vi "Pulse_Period_Measurement.vi"() -> ()   [LabVIEW 2019]
uses:
  <vilib>/Platform/TimedLoop/XDataNode/timing_clust.ctl
  <vilib>/Platform/TimedLoop/XDataNode/nitl_modes.ctl
  <vilib>/Platform/TimedLoop/XDataNode/wakeup.ctl
  <vilib>/rvi/Emulation/niFpgaSctlEmulationGetInTimedLoop.vi
  <vilib>/rvi/Emulation/niFpgaEmulationReportErrorSimple.vi
  <vilib>/rvi/Emulation/niFpgaGetClockAttributes.vi
  <vilib>/rvi/Emulation/niFpgaCriticalErrorInLSC.vi
  <vilib>/rvi/eio/common/nirviEmuTemplateMethod_errors.vi
  <vilib>/platform/TimedLoop/XDataNode/XDataNode.xnode
  <vilib>/eio/EIONode/EIONode.xnode
  <vilib>/Platform/TimedLoop/XDataNode/XDNodeRunTimeDep.lvlib
panel:
  out "DIO3_MODE_SWITCH":u32
  out "DIO2_ON_OFF_SWITCH":u32
  out "DIO1_R_THROTTLE":u32
  out "DIO0_L_THROTTLE":u32
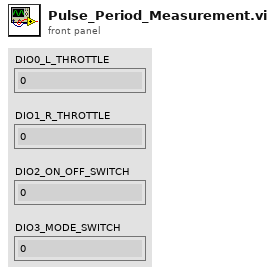
[diagram p1: front panel]
types:
  T1 = typedef "XDNodeRunTimeDep.lvlib/timing_clust.ctl" = cluster{"Expected End [f-1]":u64, "Actual End [f-1]":u64, "Finished Late? [f-1]":bool, "Expected End [i-1]":u64, "Actual End [i-1]":u64, "Finished Late? [i-1]":bool, "Expected Start [i]":u64, "Actual Start [i]":u64, "Expected Start [f]":u64, "Actual Start [f]":u64, "Source Name":string, "Structure Name":string, "Period":i64, "Deadline":i64, "Offset":i64, "Start":i64, "Priority":i32, "Timeout":i32, "Mode":T2, "Wakeup Reason":T3, "Error":errorcluster, "Source Type":string, "Secondary Source Type":string, "Global End Time":u64, "Global Start Time":u64, "Frame Duration":u64, "Iteration Duration":u64, "Assigned CPU":i32, "I/O Scan Engine Mode":u32}
  T2 = typedef "XDNodeRunTimeDep.lvlib/nitl_modes.ctl" = enum32{"No Change", "Process missed periods, maintain original phase", "Discard missed periods, maintain original phase", "Process missed periods, ignore original phase", "Discard missed periods, ignore original phase"}
  T3 = typedef "XDNodeRunTimeDep.lvlib/wakeup.ctl" = enum32{"Normal", "Aborted", "Asynchronous wakeup", "Timing source error", "Timed loop error", "Timeout"}
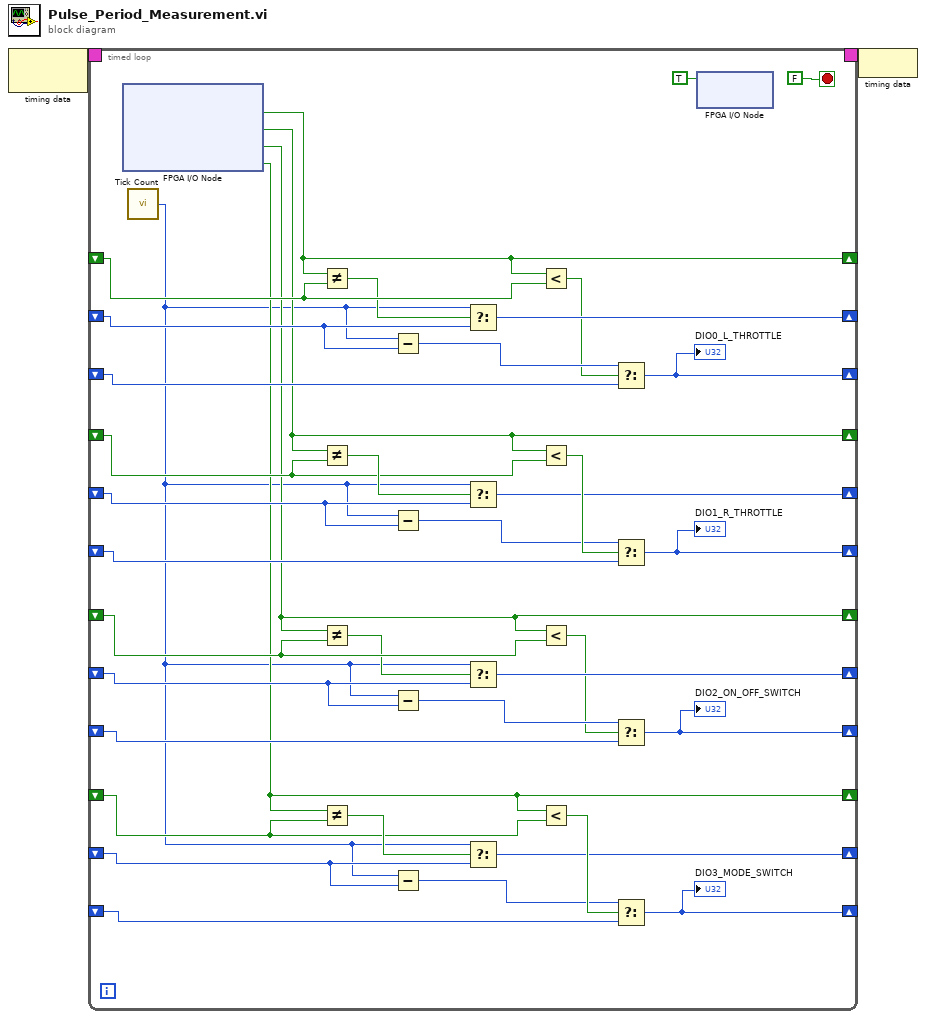
[diagram p0: block diagram]
diagram:
  n1 = node-c288() -> (w2:T1)  [unwired: 1 in]
  n2 = timed-loop {
    timing: w2 -> [_]
    timing-out: [_] -> w1
    shift-right: [w39] -> _
    shift-left: _ -> [w38]
    shift-right: [w36] -> _
    shift-left: _ -> [w35]
    shift-right: [w31] -> _
    shift-left: _ -> [w33]
    shift-right: [w6] -> _
    shift-left: _ -> [w23]
    shift-right: [w25] -> _
    shift-left: _ -> [w26]
    shift-right: [w30] -> _
    shift-left: _ -> [w28]
    shift-right: [w5] -> _
    shift-left: _ -> [w22]
    shift-right: [w20] -> _
    shift-left: _ -> [w19]
    shift-right: [w15] -> _
    shift-left: _ -> [w17]
    shift-right: [w4] -> _
    shift-left: _ -> [w7]
    shift-right: [w9] -> _
    shift-left: _ -> [w10]
    shift-right: [w14] -> _
    shift-left: _ -> [w12]
    stop <- FALSE stop-if-true
    n3 = xnode "FPGA I/O Node"() -> ("ConnectorC/DIO0"=w39:bool, "ConnectorC/DIO1"=w6:bool, "ConnectorC/DIO2"=w5:bool, "ConnectorC/DIO3"=w4:bool)  [unwired: 4 in, 4 out]
    n4 = call "Tick Count"() -> ("Tick Count(Ticks)"=w3:u32)
    n5 = Not Equal?(x=w39, y=w38) -> (x != y?=w37:bool)
    n6 = Not Equal?(x=w6, y=w23) -> (x != y?=w24:bool)
    n7 = Not Equal?(x=w5, y=w22) -> (x != y?=w21:bool)
    n8 = Not Equal?(x=w4, y=w7) -> (x != y?=w8:bool)
    n9 = Subtract(x=w3, y=w35) -> (x-y=w34:u32)
    n10 = Subtract(x=w3, y=w26) -> (x-y=w27:u32)
    n11 = Subtract(x=w3, y=w19) -> (x-y=w18:u32)
    n12 = Subtract(x=w3, y=w10) -> (x-y=w11:u32)
    n13 = Select(t=w3, s=w37, f=w35) -> (s? t:f=w36:u32)
    n14 = Select(t=w3, s=w24, f=w26) -> (s? t:f=w25:u32)
    n15 = Select(t=w3, s=w21, f=w19) -> (s? t:f=w20:u32)
    n16 = Select(t=w3, s=w8, f=w10) -> (s? t:f=w9:u32)
    n17 = Less?(x=w39, y=w38) -> (x < y?=w32:bool)
    n18 = Less?(x=w6, y=w23) -> (x < y?=w29:bool)
    n19 = Less?(x=w5, y=w22) -> (x < y?=w16:bool)
    n20 = Less?(x=w4, y=w7) -> (x < y?=w13:bool)
    n21 = Select(t=w34, s=w32, f=w33) -> (s? t:f=w31:u32)
    "DIO0_L_THROTTLE" <- w31
    n22 = Select(t=w27, s=w29, f=w28) -> (s? t:f=w30:u32)
    "DIO1_R_THROTTLE" <- w30
    n23 = Select(t=w18, s=w16, f=w17) -> (s? t:f=w15:u32)
    "DIO2_ON_OFF_SWITCH" <- w15
    n24 = Select(t=w11, s=w13, f=w12) -> (s? t:f=w14:u32)
    "DIO3_MODE_SWITCH" <- w14
    n25 = xnode "FPGA I/O Node"("LED0"=TRUE) -> ()  [unwired: 1 in, 1 out]
  }
  n26 = node-c288(w1) -> ()
